vi "Dereference Outline Glyph.vi"(8 "error in (no error)":errorcluster, 11 "glyph ref in":i64) -> (0 "error out":errorcluster, 2 "Outline Glyph Rec":T1, 3 "glyph ref out":i64)   [LabVIEW 2023, in "Freetype Drawer.lvlib"]
uses:
  Freetype Drawer.lvlib
  Outline Glyph Rec.ctl
  Glyph Rec.ctl
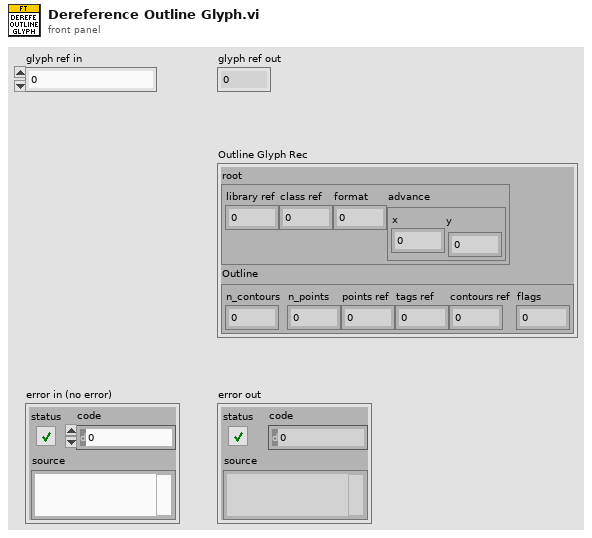
[diagram p1: front panel]
types:
  T1 = typedef "Freetype Drawer.lvlib/Outline Glyph Rec.ctl" = cluster{"root":T2, "Outline":cluster{"n_contours":i16, "n_points":i16, "points ref":i64, "tags ref":i64, "contours ref":i64, "flags":i32}}
  T2 = typedef "Freetype Drawer.lvlib/Glyph Rec.ctl" = cluster{"library ref":i64, "class ref":i64, "format":i32, "advance":cluster{"x":i32, "y":i32}}
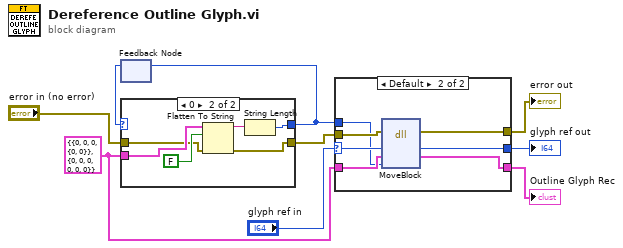
[diagram p0: block diagram]
diagram:
  w8 = T1 {"root"={"library ref"=0, "class ref"=0, "format"=0, "advance"={"x"=0, "y"=0}}, "Outline"={"n_contours"=0, "n_points"=0, "points ref"=0, "tags ref"=0, "contours ref"=0, "flags"=0}} ("Outline Glyph Rec")
  n1 = feedback #1() -> (w2:i32)  [unwired: 1 in]
  n2 = case shown="0" w2 {
    selector: w2 -> [w11 _]
    tunnel: w8 -> [_ w16]
    tunnel: "error in (no error)" -> [w10 w15]
    tunnel: [w10 w14] -> w4
    tunnel: [w11 w12] -> w1
    frame Default {
    }
    frame 0 {
      n3 = Flatten To String(anything=w16, prepend array or string size? (T)=FALSE, error in (no error)=w15) -> (data string=w13:string, error out=w14:errorcluster)  [unwired: 1 in, 1 out]
      n4 = String Length(string=w13) -> (length=w12:i32)
    }
  }
  n5 = feedback-in #1(w1) -> ()
  n6 = case shown="Default" "glyph ref in" {
    selector: "glyph ref in" -> [w19 w24]
    tunnel: [w20 w27] -> w9
    tunnel: w8 -> [w18 w26]
    tunnel: [w19 w25] -> w7
    tunnel: w4 -> [w20 w23]
    tunnel: w1 -> [_ w22]
    tunnel: [w18 w21] -> w3
    frame 0 {
    }
    frame Default {
      n7 = dll-call lib="LabVIEW" fn="MoveBlock"(error in=w23, "in"=w24, "out"=w26, "size"=w22) -> (error out=w27:errorcluster, "in"=w25:i64, "out"=w21:T1)  [unwired: 4 in, 1 out]
    }
  }
  "error out" <- w9
  "glyph ref out" <- w7
  "Outline Glyph Rec" <- w3
